vi "System Saftey Monitoring Loop.vi"(8 "error in (no error)":errorcluster, 9 "System Data Display Ref":refnum<vi>, 10 "Data Queue":refnum<queue>, 11 "Message Queues":T1) -> (0 "error out":errorcluster)   [LabVIEW 2026]
uses:
  support/Message Queue/All Message Queues.ctl
  support/Message Queue/Message Cluster.ctl
  Acquisition/Hardware Configuration.ctl
  Acquisition/Acquisition State.ctl
  <vilib>/DAQmx/read.llb/DAQmx Read (Digital 1D Bool NChan 1Samp 1Line).vi
  support/Message Queue/Enqueue Message (Single).vi
  <vilib>/DAQmx/miscellaneous.llb/DAQmx Fill In Error Info.vi
  <vilib>/Utility/error.llb/Error Cluster From Error Code.vi
  <vilib>/ErrorRing/Error Ring.xnode
  Acquisition/Acquisition.lvlib
  support/Message Queue/Message Queue.lvlib
  controls/Abort.vi
panel:
  out "Table Control":string[][](table)
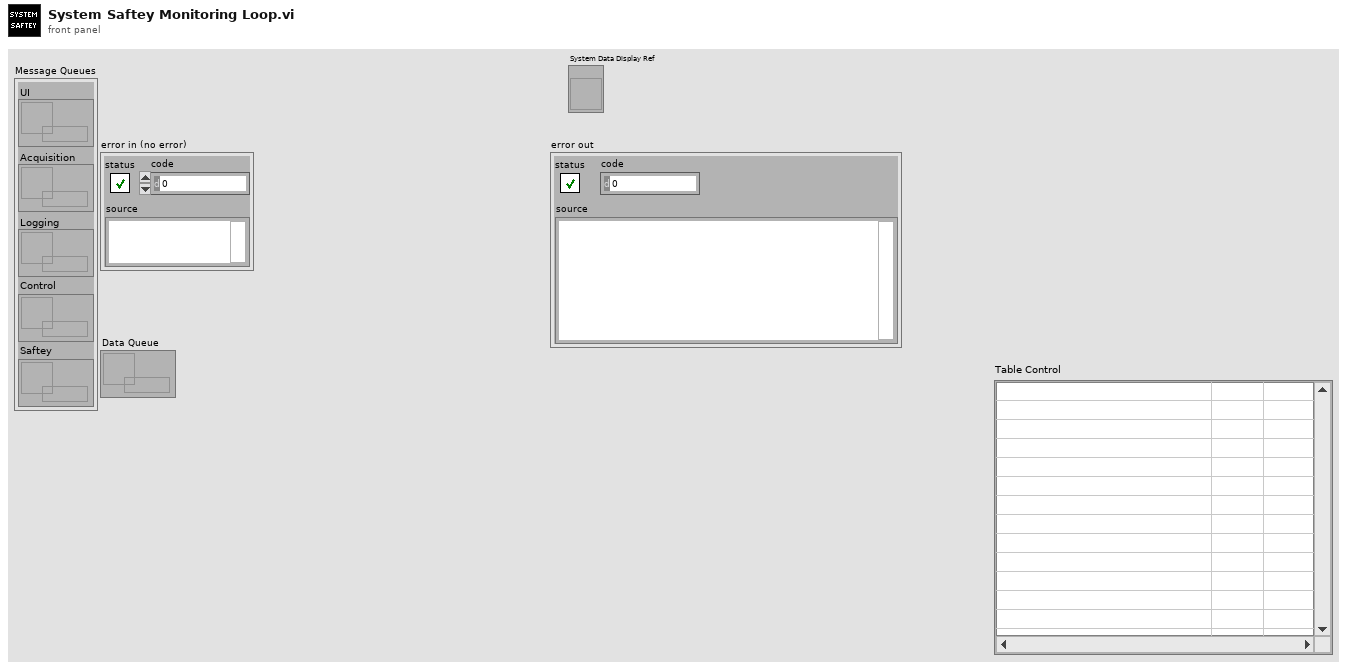
[diagram p1: front panel]
types:
  T1 = typedef "Message Queue.lvlib/All Message Queues.ctl" = cluster{"UI":refnum<queue>, "Acquisition":refnum<queue>, "Logging":refnum<queue>, "Control":refnum<queue>, "Saftey":refnum<queue>}
  T2 = typedef "Acquisition.lvlib/Hardware Configuration.ctl" = cluster{"Analog Out array":dbl[], "Initialize Flag":bool, "Saftey Table Display":refnum<vi>, "Torque&Force":waveform(dbl)[][], "Calibration Data":waveform(dbl)[], "2D":dbl[][], "Analog In Task":refnum<k21>, "Digital In Task":refnum<k21>, "Analog Out Task":refnum<k21>, "Digital Out Task":refnum<k21>, "Digital Out Array":bool[], "Current Cycle Count":refnum<vi>, "Cycle Count":u64, "Headers":string[], "Sweep Interval":u64, "Delay":u64, "TestConfigDisplay":refnum<vi>, "50psi Conversion":dbl[], "1245N15 Conversion":dbl[], "MX06F Conversion":dbl[], "# of Test Cycles":u64, "60psi Conversion":dbl[], "100psi Conversion":dbl[], "200psi Conversion":dbl[], "1000psi Conversion":dbl[], "2000psi Conversion":dbl[], "5000psi Conversion":dbl[], "MX09F Conversion":dbl[], "MX19F Conversion":dbl[]}
  T3 = typedef "Acquisition.lvlib/Acquisition State.ctl" = enum16{"Idle", "Acquiring"}
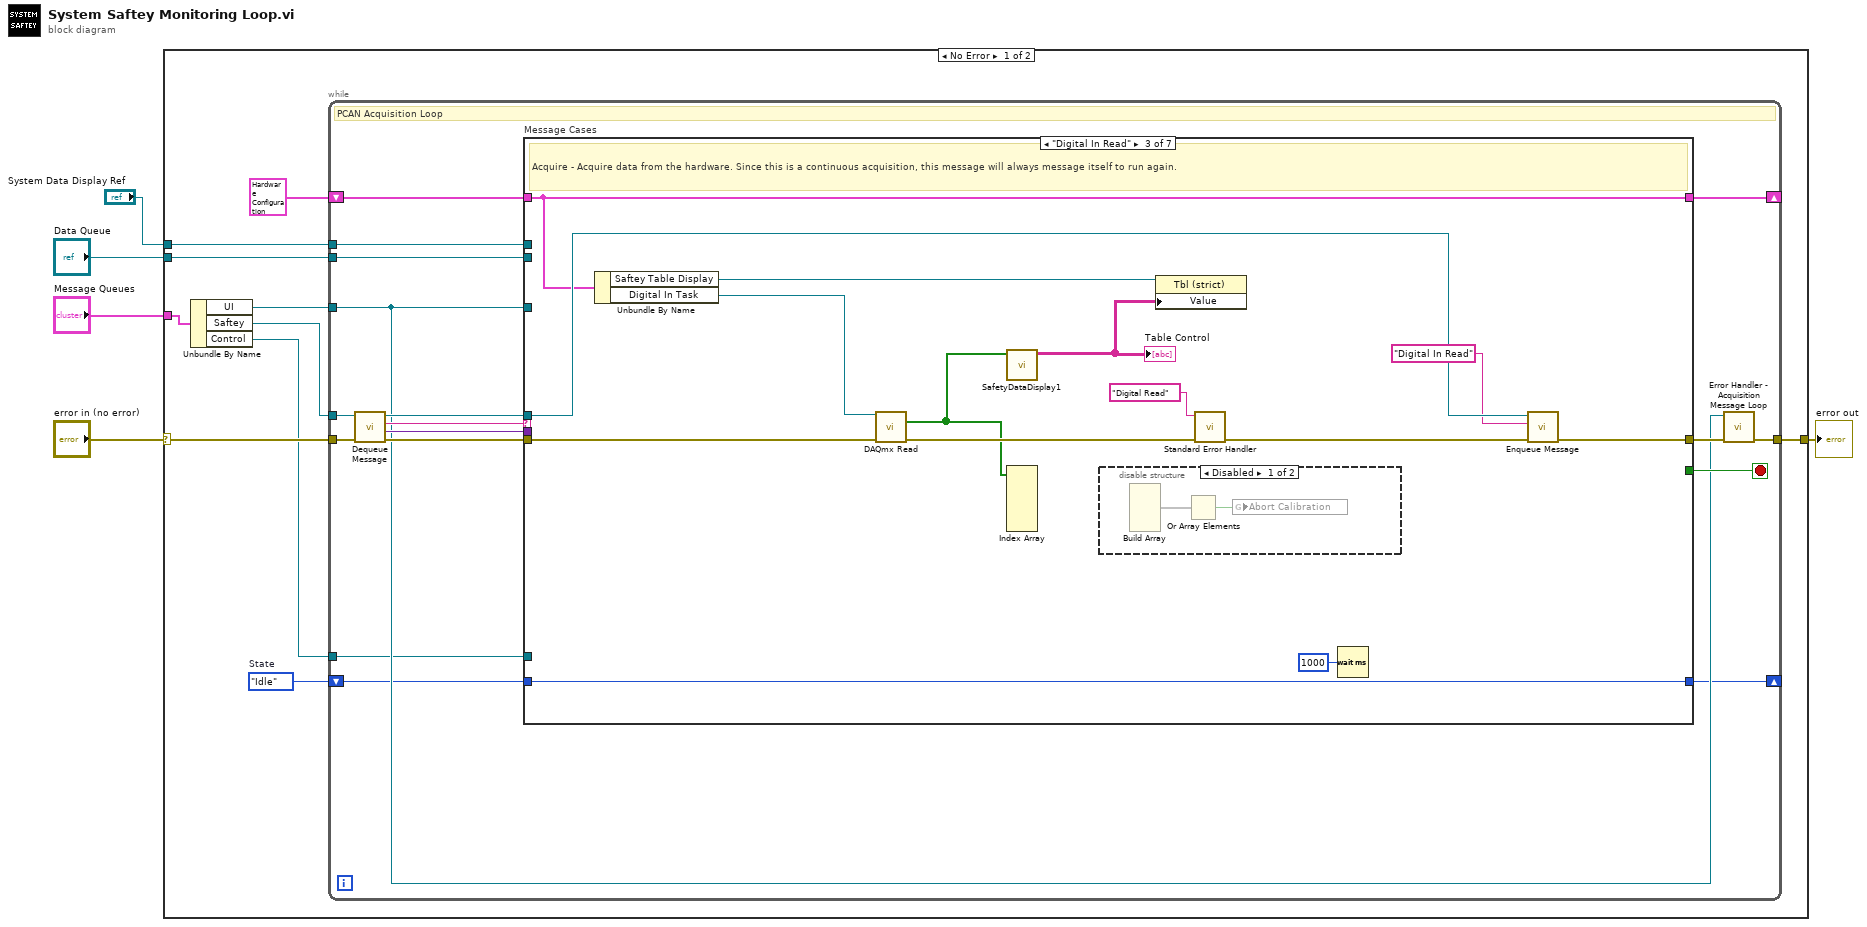
[diagram p0: block diagram]
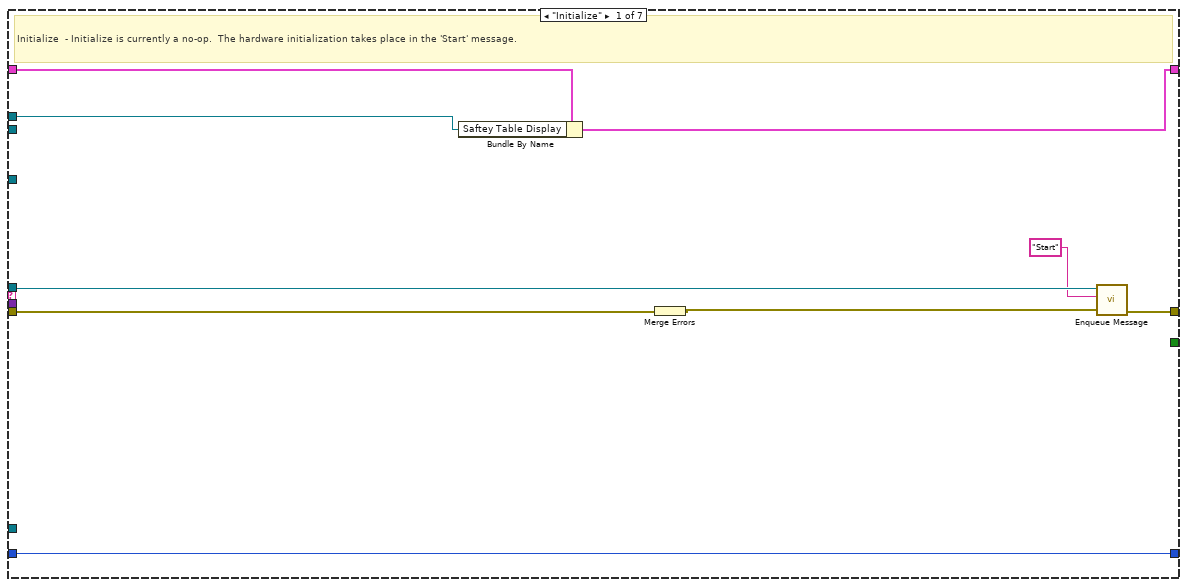
[diagram p2: hidden frame]
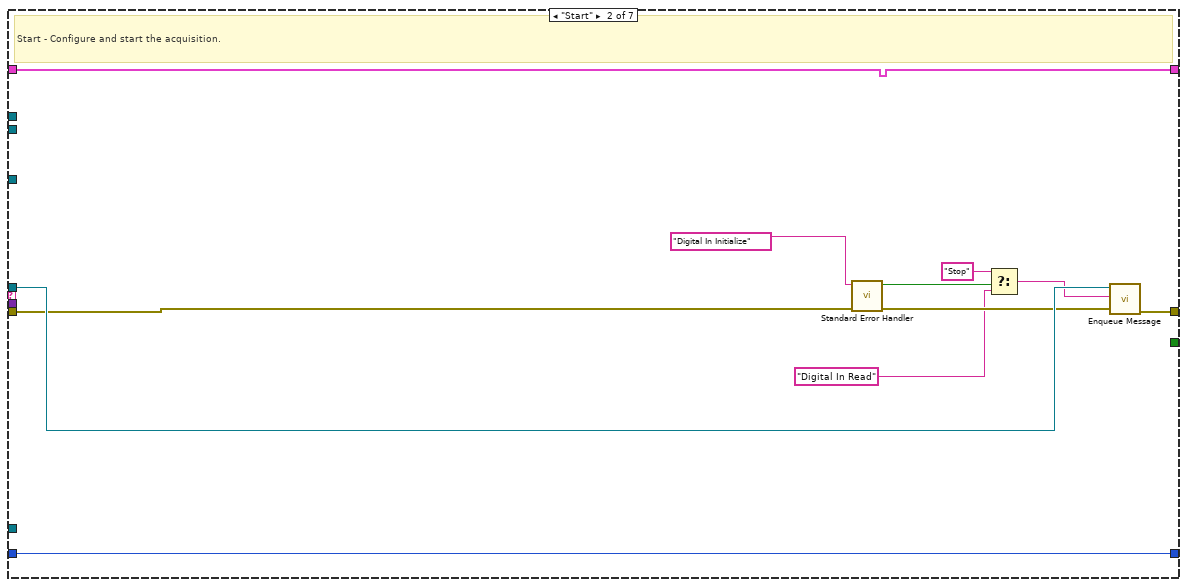
[diagram p3: hidden frame]
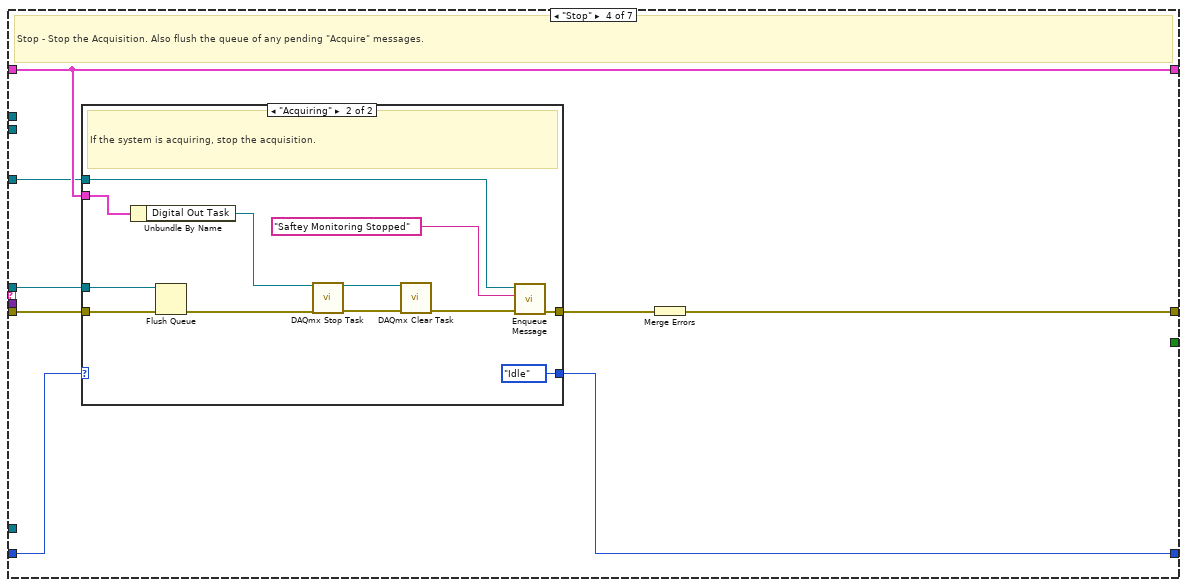
[diagram p5: hidden frame]
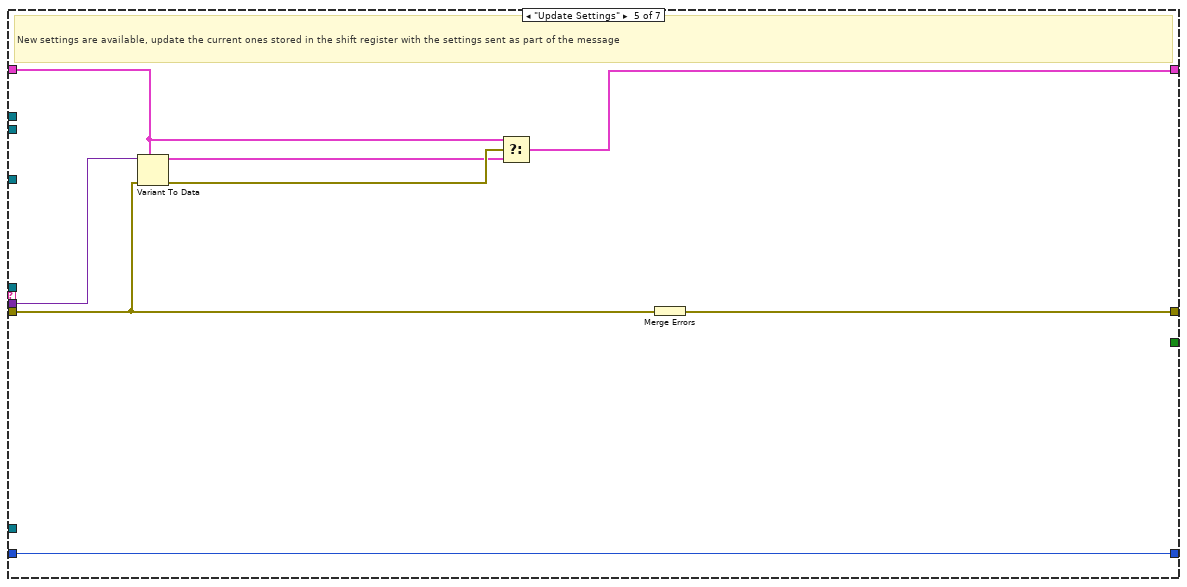
[diagram p7: hidden frame]
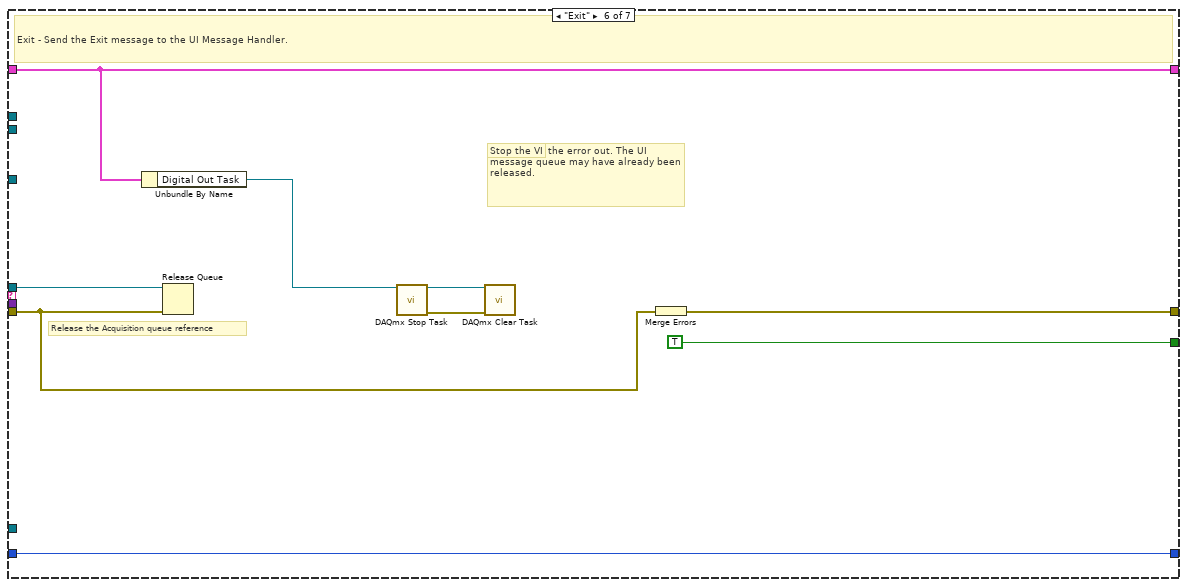
[diagram p8: hidden frame]
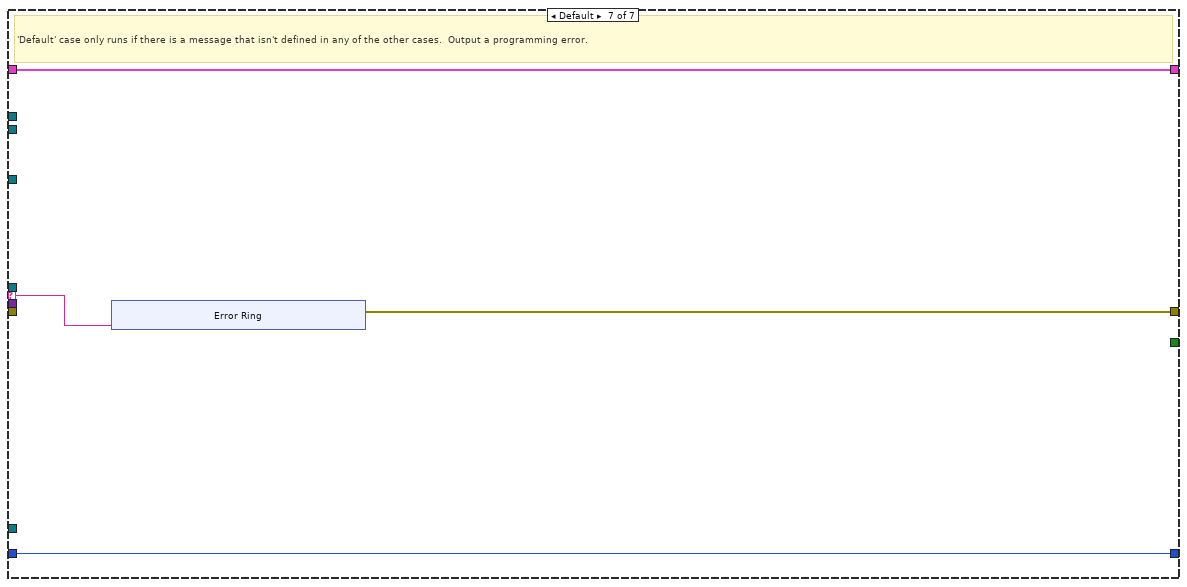
[diagram p9: hidden frame]
diagram:
  n1 = case shown="No Error" "error in (no error)" {
    selector: "error in (no error)" -> [w12 w119]
    tunnel: "Message Queues" -> [w15 _]
    tunnel: [w14 w119] -> w4
    tunnel: "Data Queue" -> [w10 _]
    tunnel: "System Data Display Ref" -> [w6 _]
    frame No Error {
      w9 = Acquisition_State."Idle"  # State
      n2 = Unbundle By Name(w15) -> ("UI"=w11:refnum<queue>, "Saftey"=w7:refnum<queue>, "Control"=w8:refnum<queue>)
      n3 = while {
        tunnel: w7 -> [w24]
        shift-right: [w31] -> _
        shift-left: T2 {"Analog Out array"=[], "Initialize Flag"=FALSE, "Saftey Table Display"=refnum, "Torque&Force"=[], "Calibration Data"=[], "2D"=[], "Analog In Task"="", "Digital In Task"="", "Analog Out Task"="", "Digital Out Task"="", "Digital Out Array"=[], "Current Cycle Count"=refnum, "Cycle Count"=0, "Headers"=[], "Sweep Interval"=0, "Delay"=0, "TestConfigDisplay"=refnum, "50psi Conversion"=[], "1245N15 Conversion"=[], "MX06F Conversion"=[], "# of Test Cycles"=0, "60psi Conversion"=[], "100psi Conversion"=[], "200psi Conversion"=[], "1000psi Conversion"=[], "2000psi Conversion"=[], "5000psi Conversion"=[], "MX09F Conversion"=[], "MX19F Conversion"=[]} ("Data Cluster") -> [w32]
        tunnel: w11 -> [w20]
        tunnel: w10 -> [w23]
        shift-right: [w18] -> _
        shift-left: w9 -> [w19]
        tunnel: w8 -> [w17]
        tunnel: w12 -> [w29]
        tunnel: [w21] -> w14
        tunnel: w6 -> [w16]
        stop <- w30 stop-if-true
        # "PCAN Acquisition Loop"
        n4 = call "Dequeue Message.vi"("error in (no error)"=w29, "Message Queue"=w24) -> ("error out"=w28:errorcluster, "Message Data"=w26:variant, "Message"=w27:string, "dup Message Queue"=w25:refnum<queue>)  [unwired: 6 in]
        n5 = case "Message Cases" shown="\"Digital In Read\"" w27 {
          selector: w27 -> [_ _ _ _ _ _ w110]
          tunnel: w25 -> [w37 w50 w65 w73 _ w105 _]
          tunnel: w28 -> [w41 w43 w59 w75 w92 w99 _]
          tunnel: [w39 w51 w64 w76 w98 w106 w109] -> w22
          tunnel: w32 -> [w35 w42 w56 w74 w94 w103 w111]
          tunnel: [w34 w42 w56 w74 w93 w103 w111] -> w31
          tunnel: [_ _ _ _ _ TRUE _] -> w30
          tunnel: w26 -> [_ _ _ _ w97 _ _]
          tunnel: w20 -> [_ _ _ w72 _ _ _]
          tunnel: w23 -> [_ _ _ _ _ _ _]
          tunnel: w19 -> [w40 w52 w66 w71 w91 w104 w108]
          tunnel: [w40 w52 w66 w70 w91 w104 w108] -> w18
          tunnel: w17 -> [_ _ _ _ _ _ _]
          tunnel: w16 -> [w33 _ _ _ _ _ _]
          frame "Initialize" {
            # "Initialize  - Initialize is currently a no-op.  The hardware initialization takes place in the 'Start' message."
            n6 = Bundle By Name(cluster=w35, "Saftey Table Display"=w33) -> (w34:T2)
            n7 = Merge Errors(w41) -> (w38:errorcluster)
            n8 = call-poly "Enqueue Message.vi"("error in (no error)"=w38, "Message"="Start" ("t"), "Message Queue"=w37) -> ("error out"=w39:errorcluster)  [unwired: 7 in, 1 out]
          }
          frame "Start" {
            # "Start - Configure and start the acquisition."
            n9 = call "Standard Error Handler.vi"("error in (no error)"=w43, "source"="Digital In Initialize") -> ("error out"=w49:errorcluster, "error?"=w48:bool)  [unwired: 8 in]
            n10 = Select(t="Stop", s=w48, f="Digital In Read") -> (s? t:f=w47:string)
            n11 = call-poly "Enqueue Message.vi"("error in (no error)"=w49, "Message"=w47, "Message Queue"=w50) -> ("error out"=w51:errorcluster)  [unwired: 7 in, 1 out]
          }
          frame "Digital In Read" {
            # "Acquire - Acquire data from the hardware. Since this is a continuous acquisition, this message will always message itself to run again."
            n12 = Unbundle By Name(w56) -> ("Saftey Table Display"=w54:refnum<vi>, "Digital In Task"=w57:refnum<k21>)
            n13 = call-poly <vilib>:"DAQmx Read.vi"("task/channels in"=w57, "error in"=w59) -> ("data"=w53:bool[], "error out"=w58:errorcluster)  [unwired: 11 in, 1 out]
            n14 = call "SafetyDataDisplay1.vi"("data"=w53) -> ("Table Control"=w55:string[][])  [unwired: 10 in]
            "Table Control" <- w55
            n15 = Index Array(array=w53) -> ()  [unwired: 6 in, 6 out]
            n16 = disable-structure shown="Disabled" {
              frame Disabled {
                n17 = Build Array() -> (w68:void[])  [unwired: 6 in]
                n18 = Or Array Elements(Boolean array=w68) -> (logical OR=w67:bool)
                n19 = global write "Abort.vi" "Abort Calibration"(w67) -> ()
              }
              frame Enabled {
              }
            }
            n20 = property class="Tbl (strict)"(reference=w54, "Value"=w55) -> ()  [unwired: 1 in, 2 out]
            n21 = call "Standard Error Handler.vi"("error in (no error)"=w58, "source"="Digital Read") -> ("error out"=w61:errorcluster)  [unwired: 8 in, 1 out]
            n22 = Wait (ms)(milliseconds to wait=u32 1000) -> ()  [unwired: 1 out]
            n23 = call-poly "Enqueue Message.vi"("error in (no error)"=w61, "Message"="Digital In Read", "Message Queue"=w65) -> ("error out"=w64:errorcluster)  [unwired: 7 in, 1 out]
          }
          frame "Stop" {
            # "Stop - Stop the Acquisition. Also flush the queue of any pending \"Acquire\" messages."
            n24 = case shown="\"Acquiring\"" w71 {
              selector: w71 -> [w78 _]
              tunnel: w75 -> [w77 w90]
              tunnel: w74 -> [_ w84]
              tunnel: w73 -> [_ w89]
              tunnel: w72 -> [_ w88]
              tunnel: [w78 Acquisition_State."Idle" ("State")] -> w70
              tunnel: [w77 w87] -> w69
              frame "Idle", Default {
                # "The system is already idle. Ignore the \"Stop\" message."
              }
              frame "Acquiring" {
                # "If the system is acquiring, stop the acquisition."
                n25 = Unbundle By Name(w84) -> ("Digital Out Task"=w81:refnum<k21>)
                n26 = Flush Queue(queue=w89, error in (no error)=w90) -> (error out=w80:errorcluster)  [unwired: 2 out]
                n27 = call <vilib>:"DAQmx Stop Task.vi"("task/channels in"=w81, "error in"=w80) -> ("task out"=w83:refnum<k21>, "error out"=w82:errorcluster)  [unwired: 12 in]
                n28 = call <vilib>:"DAQmx Clear Task.vi"("task in"=w83, "error in"=w82) -> ("error out"=w79:errorcluster)  [unwired: 13 in]
                n29 = call-poly "Enqueue Message.vi"("error in (no error)"=w79, "Message"="Saftey Monitoring Stopped", "Message Queue"=w88) -> ("error out"=w87:errorcluster)  [unwired: 7 in, 1 out]
              }
            }
            n30 = Merge Errors(w69) -> (w76:errorcluster)
          }
          frame "Update Settings" {
            # "New settings are available, update the current ones stored in the shift register with the settings sent as part of the message"
            n31 = Variant To Data(error in=w92, type=w94, Variant=w97) -> (data=w95:T2, error out=w96:errorcluster)
            n32 = Select(t=w94, s=w96, f=w95) -> (s? t:f=w93:T2)
            n33 = Merge Errors(w92) -> (w98:errorcluster)
          }
          frame "Exit" {
            # "Don't check the error out. The UI message queue may have already been released."
            # "Release the Acquisition queue reference"
            # "Stop the VI"
            # "Exit - Send the Exit message to the UI Message Handler."
            n34 = Unbundle By Name(w103) -> ("Digital Out Task"=w100:refnum<k21>)
            n35 = Release Queue(queue=w105, error in (no error)=w99) -> ()  [unwired: 1 in, 3 out]
            n36 = call <vilib>:"DAQmx Stop Task.vi"("task/channels in"=w100) -> ("task out"=w102:refnum<k21>, "error out"=w101:errorcluster)  [unwired: 13 in]
            n37 = call <vilib>:"DAQmx Clear Task.vi"("task in"=w102, "error in"=w101) -> ()  [unwired: 13 in, 1 out]
            n38 = Merge Errors(w99) -> (w106:errorcluster)
          }
          frame Default {
            # "'Default' case only runs if there is a message that isn't defined in any of the other cases.  Output a programming error."
            n39 = xnode "Error Ring"("parameter 0"=w110) -> ("error out"=w109:errorcluster)
          }
        }
        n40 = call "Error Handler - Acquisition Message Loop.vi"("error in (no error)"=w22, "Message Queue"=w20) -> ("dup error in"=w21:errorcluster)  [unwired: 8 in, 1 out]
      }
    }
    frame Error {
    }
  }
  "error out" <- w4
